vi "URL Write 3.vi"(4 "error in (no error)":errorcluster, 5 "Value":string, 6 "Container State":T3, 7 "Display State In":T1={"WebView2 Ref"=refnum, "event callback refnum"=refnum, "Events"={"Navigation Complete Event"=refnum, "Source Changed Event"=refnum, "Document Title Changed Event"=refnum, "Status Bar Text Changed"=refnum, "Web Message Received"=refnum, "Window Close Requested"=refnum}, "Paths"={"Webview2 Native"=path "C:/Users/kleins/Desktop/webview2/microsoft.web.webview2.1.0.1370.28/build/native", "Edge Application"=path "", "User Data"=path ""}}) -> (0 "error out":errorcluster, 3 "Display State Out":T1={"WebView2 Ref"=refnum, "event callback refnum"=refnum, "Events"={"Navigation Complete Event"=refnum, "Source Changed Event"=refnum, "Document Title Changed Event"=refnum, "Status Bar Text Changed"=refnum, "Web Message Received"=refnum, "Window Close Requested"=refnum}, "Paths"={"Webview2 Native"=path "C:/Users/kleins/Desktop/webview2/microsoft.web.webview2.1.0.1370.28/build/native", "Edge Application"=path "", "User Data"=path ""}})   [LabVIEW 2020, in "WebView2 Control.xctl"]
uses:
  WebView2 Control.xctl
  <vilib>/_xctls/Container State.ctl
  State.ctl
  C:/Users/kleins/Desktop/webview2/microsoft.web.webview2.1.0.1370.28/lib/net45/Microsoft.Web.WebView2.WinForms.dll
  microsoft.web.webview2.1.0.1370.28/lib/net45/Microsoft.Web.WebView2.WinForms.dll
  Paths.ctl
  C:/Users/kleins/Desktop/webview2/microsoft.web.webview2.1.0.1370.28/lib/net45/Microsoft.Web.WebView2.Core.dll
  microsoft.web.webview2.1.0.1370.28/lib/net45/Microsoft.Web.WebView2.Core.dll
  <vilib>/_xctls/XControlSupport.lvlib
panel:
  # "Replace the Value Control below with a Control of desired type.\nDo not remove this Control or the others from the connector pane.\nDo not change the connector pane pattern.\nThe Value control should always be the third terminal from top on the input side in the connector pane."
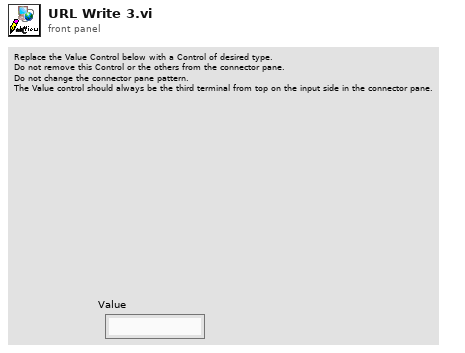
[diagram p1: front panel]
types:
  T1 = typedef "WebView2 Control.xctl/State.ctl" = cluster{"WebView2 Ref":refnum<data-value>, "event callback refnum":refnum<k27>, "Events":cluster{"Navigation Complete Event":refnum<user-event>, "Source Changed Event":refnum<user-event>, "Document Title Changed Event":refnum<user-event>, "Status Bar Text Changed":refnum<user-event>, "Web Message Received":refnum<user-event>, "Window Close Requested":refnum<user-event>}, "Paths":T2}
  T2 = typedef "WebView2 Control.xctl/Paths.ctl" = cluster{"Webview2 Native":path, "Edge Application":path, "User Data":path}
  T3 = typedef "XControlSupport.lvlib/Container State.ctl" = cluster{"Indicator?":bool, "Run Mode?":bool, " Refnum":refnum<vi>}
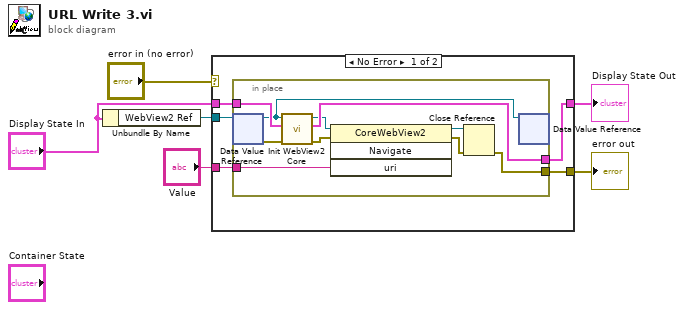
[diagram p0: block diagram]
diagram:
  n1 = Unbundle By Name("Display State In") -> ("WebView2 Ref"=w6:refnum<data-value>)
  n2 = case shown="No Error" "error in (no error)" {
    selector: "error in (no error)" -> [_ w23]
    tunnel: [w11 w23] -> w4
    tunnel: w6 -> [w10 _]
    tunnel: "Value" -> [w9 _]
    tunnel: "Display State In" -> [w8 w22]
    tunnel: [w7 w22] -> w1
    frame No Error {
      n3 = in-place {
        in-place-border: [w18] -> w11
        in-place-border: w9 -> [w20]
        in-place-border: w8 -> [w17]
        in-place-border: [w16] -> w7
        n4 = in-place-dvr #1(w10) -> (w12:refnum<k24>, w14:errorcluster)
        n5 = call "Init WebView2 Core.vi"("error in (no error)"=w14, "Display State In"=w17, ".NET Refnum in"=w12) -> ("error out"=w13:errorcluster, "Display State In 2"=w16:T1, ".NET Refnum out"=w15:refnum<k24>)  [unwired: 6 in]
        n6 = invoke class="CoreWebView2" method="Navigate"(reference=w15, error in=w13, "uri"=w20) -> (reference out=w19:refnum<k24>, error out=w21:errorcluster)  [unwired: 1 in, 2 out]
        n7 = Close Reference(reference=w19, error in (no error)=w21) -> (error out=w18:errorcluster)
        n8 = in-place-dvr #1(w12) -> ()  [unwired: 2 out]
      }
    }
    frame Error {
    }
  }
  "error out" <- w4
  "Display State Out" <- w1
